vi "Local Dispatch Loop.vi"(11 "TCPMessaging in":refnum<class "TCPMessaging.lvclass">) -> ()   [LabVIEW 2020, in "Vecto.lvlib" / "TCPMessaging.lvclass"]
uses:
  TCPMessaging.lvclass
  TCPMessaging.lvclass/TCPMessaging.ctl
  TCPMessageHandler/TCPMessageHandler.lvclass
  proto/TcpPayload/TcpPayload.lvlib
  proto/TcpClientList/TcpClientList.lvlib
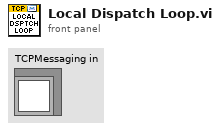
[diagram p1: front panel]
types:
  T1 = typedef "TcpPayload.lvlib/Data.ctl" = cluster{"target_node":u32, "source_id":u32, "sequence":u32, "timestamp":i64, "type":string, "task_id":string, "payload":u8[]}
  T2 = typedef "TcpClientList.lvlib/Data.ctl" = cluster{"clients":T3[]}
  T3 = typedef "TcpClientInfo.lvlib/Data.ctl" = cluster{"node_id":u32, "node_name":string, "app_version":string, "config_version":string, "config_hash":string, "node_alias":string, "address":string}
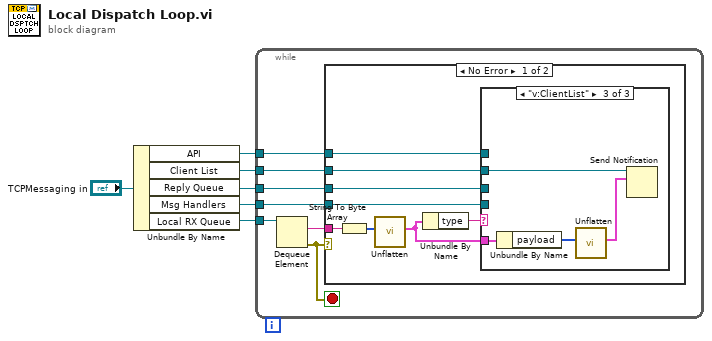
[diagram p0: block diagram]
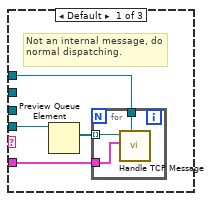
[diagram p2: hidden frame]
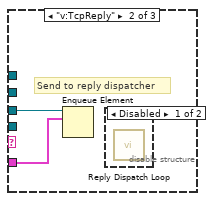
[diagram p3: hidden frame]
diagram:
  n1 = Unbundle By Name("TCPMessaging in") -> ("API"=w1:refnum<class "TCPMessageAPI.lvclass">, "Client List"=w2:refnum<notifier>, "Reply Queue"=w3:refnum<queue>, "Msg Handlers"=w5:refnum<queue>, "Local RX Queue"=w6:refnum<queue>)
  n2 = while {
    tunnel: w6 -> [w13]
    tunnel: w5 -> [w12]
    tunnel: w1 -> [w10]
    tunnel: w3 -> [w8]
    tunnel: w2 -> [w7]
    stop <- w9 stop-if-true
    n3 = Dequeue Element(queue=w13) -> (element=w11:string, error out=w9:errorcluster)  [unwired: 2 in, 2 out]
    n4 = case shown="No Error" w9 {
      tunnel: w12 -> [w21 _]
      tunnel: w11 -> [w20 _]
      tunnel: w10 -> [w18 _]
      tunnel: w8 -> [w15 _]
      tunnel: w7 -> [w14 _]
      frame No Error {
        n5 = String To Byte Array(string=w20) -> (unsigned byte array=w19:u8[])
        n6 = call "Unflatten.vi"("Buffer"=w19) -> ("Data"=w17:T1)  [unwired: 9 in, 1 out]
        n7 = Unbundle By Name(w17) -> ("type"=w16:string)
        n8 = case shown="\"v:ClientList\"" w16 {
          tunnel: w21 -> [w25 _ _]
          tunnel: w18 -> [w23 _ _]
          tunnel: w17 -> [w22 w29 w34]
          tunnel: w15 -> [_ w30 _]
          tunnel: w14 -> [_ _ w32]
          frame Default {
            # "Not an internal message, do normal dispatching."
            n9 = Preview Queue Element(queue=w25) -> (element=w24:refnum<class "TCPMessageHandler.lvclass">[])  [unwired: 2 in, 3 out]
            n10 = for {
              tunnel: w24 -> [w28] mode=indexing
              tunnel: w23 -> [w27]
              tunnel: w22 -> [w26]
              n11 = call-dynamic "Handle TCP Message.vi"("TCPMessageAPI"=w27, "TcpPayload"=w26, "TCPMessageHandler in"=w28) -> ()  [unwired: 7 in, 2 out]
            }
          }
          frame "v:TcpReply" {
            # "Send to reply dispatcher"
            n12 = Enqueue Element(queue=w30, element=w29) -> ()  [unwired: 2 in, 3 out]
            n13 = disable-structure shown="Disabled" {
              frame Disabled {
                n14 = call "Reply Dispatch Loop.vi"() -> ()  [unwired: 11 in, 1 out]
              }
              frame Enabled {
              }
            }
          }
          frame "v:ClientList" {
            n15 = Unbundle By Name(w34) -> ("payload"=w33:u8[])
            n16 = call "Unflatten.vi"("Buffer"=w33) -> ("Data"=w31:T2)  [unwired: 9 in, 1 out]
            n17 = Send Notification(notification=w31, notifier=w32) -> ()  [unwired: 1 in, 2 out]
          }
        }
      }
      frame Error {
      }
    }
  }
